vi "Option Parser.vi"(0 "Yokogawa WT500 in":refnum<class "Yokogawa WT500.lvclass">, 1 "ID":string, 2 "THD?":bool, 3 "Number of Cards":dbl, 4 "ID cluster.Model":string, 5 "error in (no error)":errorcluster, 7 "Option":string) -> (14 "Yokogawa WT500 out":refnum<class "Yokogawa WT500.lvclass">, 19 "error out":errorcluster)   [LabVIEW 2014, in "Generic Power Analyzer.lvlib" / "Yokogawa WT500.lvlib" / "Yokogawa WT500.lvclass"]
uses:
  Yokogawa WT500.lvclass
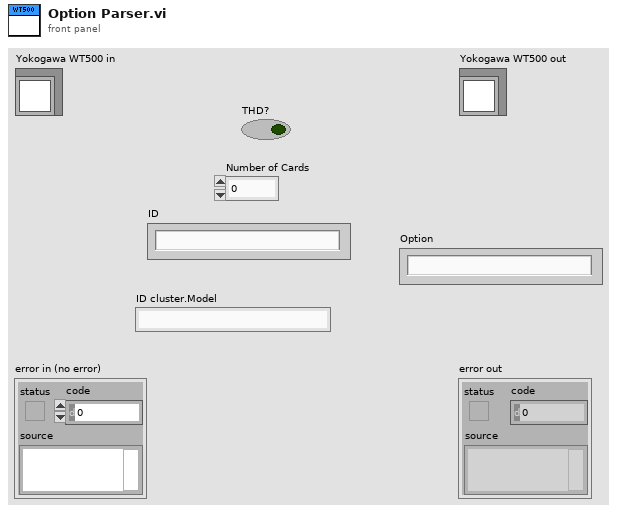
[diagram p1: front panel]
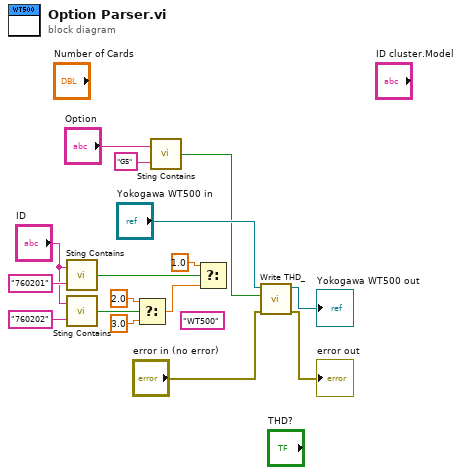
[diagram p0: block diagram]
diagram:
  (unwired) "WT500" ("ID cluster.Model")
  n1 = call "Sting Contains.vi"("Expression to evaluate"="760201", "Input String"="ID") -> ("Boolean"=w13:bool)
  n2 = call "Sting Contains.vi"("Expression to evaluate"="760202", "Input String"="ID") -> ("Boolean"=w9:bool)
  n3 = Select(t=2.0, s=w9, f=3.0) -> (s? t:f=w8:dbl)
  n4 = call "Sting Contains.vi"("Expression to evaluate"="G5", "Input String"="Option") -> ("Boolean"=w3:bool)
  n5 = Select(t=1.0, s=w13, f=w8) -> ()  [unwired: 1 out]
  n6 = call-dynamic "Write THD_.vi"("error in (no error)"="error in (no error)", "THD?"=w3, "Generic Power Analyzer in"="Yokogawa WT500 in") -> ("error out"=→"error out":errorcluster, "Generic Power Analyzer out"=→"Yokogawa WT500 out":refnum<class "Yokogawa WT500.lvclass">)  [unwired: 7 in]
